vi "table sort by column.vi"(9 "Column to sort":i32, 10 "Sorting Type":T1, 11 "Array":string[][](array[string])) -> (3 "sorted array":string[][](array[string]))   [LabVIEW 2013, in "PL Framework Configuration Tool.lvlib" / "Engine Mappings.lvclass"]
uses:
  Engine Mappings.lvclass
  mapping sort type.ctl
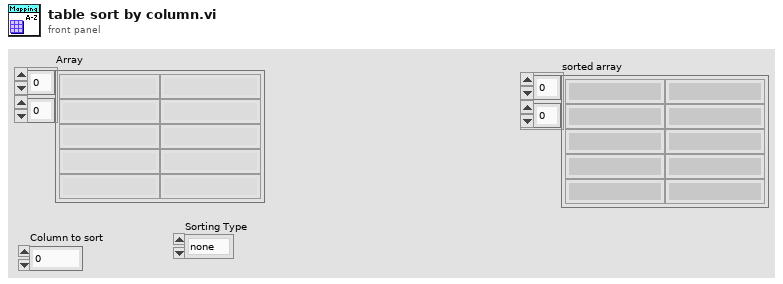
[diagram p1: front panel]
types:
  T1 = typedef "PL Framework Configuration Tool.lvlib/Engine Mappings.lvclass/mapping sort type.ctl" = enum16{"none", "asc", "desc"}
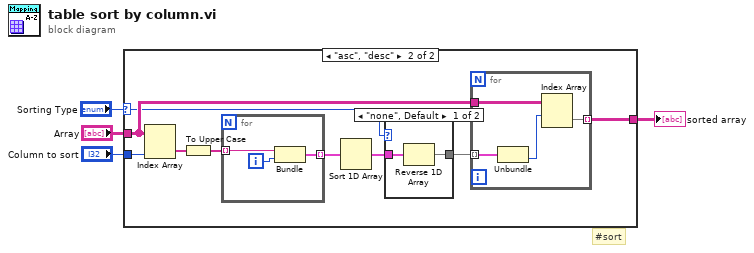
[diagram p0: block diagram]
diagram:
  # "#sort"
  n1 = case shown="\"asc\", \"desc\"" "Sorting Type" {
    selector: "Sorting Type" -> [_ w8]
    tunnel: "Column to sort" -> [_ w14]
    tunnel: "Array" -> [w5 w12]
    tunnel: [w5 w9] -> w2
    frame "none" {
    }
    frame "asc", "desc" {
      n2 = Index Array(array=w12, index (col)=w14) -> (element=w11:string[])  [unwired: 1 in]
      n3 = To Upper Case(1:w11) -> (0:w10:string[])
      n4 = for {
        tunnel: w10 -> [w24] mode=indexing
        tunnel: [w22] -> w13 mode=indexing
        i -> [w23]
        n5 = Bundle("String"=w24, w23) -> (w22:cluster{"String":string, i32})  [unwired: 1 in]
      }
      n6 = Sort 1D Array(array=w13) -> (sorted array=w6:cluster{"String":string, i32}[])
      n7 = case shown="\"none\", Default" w8 {
        tunnel: [w15 w17] -> w7
        tunnel: w6 -> [w16 w17]
        frame "none", Default {
          n8 = Reverse 1D Array(array=w16) -> (reversed array=w15:cluster{"String":string, i32}[])
        }
        frame "asc" {
        }
      }
      n9 = for {
        tunnel: w12 -> [w19]
        tunnel: w7 -> [w21] mode=indexing
        tunnel: [w18] -> w9 mode=indexing
        n10 = Unbundle(w21) -> (w20:i32)  [unwired: 1 out]
        n11 = Index Array(array=w19, index (row)=w20) -> (element=w18:string[])  [unwired: 1 in]
      }
    }
  }
  "sorted array" <- w2
